vi "Test50.vi"(0 "L2T":T1 caption="Limites de test pris en compte", 2 "SN":string="0B5MEVA000CA1JC1M0000041", 3 "errin":errorcluster, 5 "Peak":T2=enum."PCAN_USBBUS1") -> (7 "RequetSQL":string, 8 "v1":string, 10 "errout":errorcluster)   [LabVIEW 2020]
uses:
  <userlib>/PCAN Basic/Controls/Channel.ctl
  Ctrl/L2T.ctl
  VarGLO/Global var.vi
  <vilib>/regexp/Match Regular Expression.xnode
  <userlib>/PCAN Basic/PCANBasic.lvlib
panel:
  out "cluster de sortie":T3
  # "Pre DCIR_____________________________________"
  # "intra DCIR_____________________________________"
  # "Post DCIR_____________________________________"
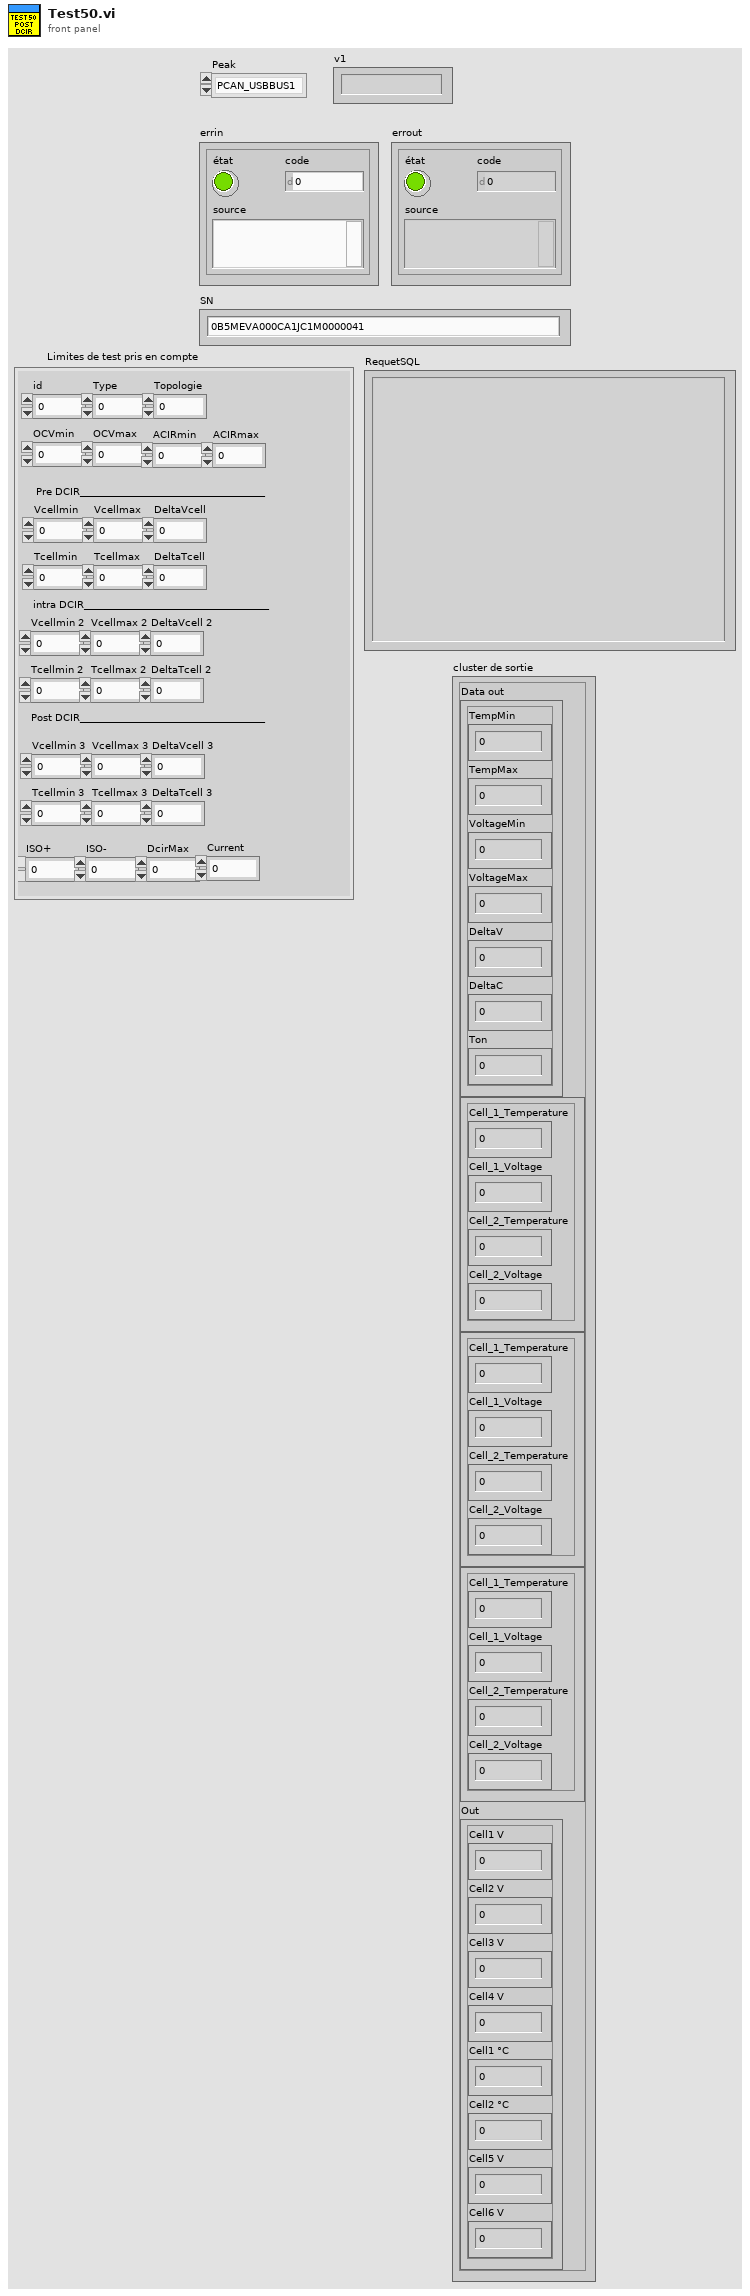
[diagram p1: front panel]
types:
  T1 = typedef "L2T.ctl" = cluster{"id":dbl, "Type":dbl, "OCVmin":dbl, "OCVmax":dbl, "ACIRmin":dbl, "ACIRmax":dbl, "Vcellmin":dbl, "Vcellmax":dbl, "DeltaVcell":dbl, "Tcellmin":dbl, "Tcellmax":dbl, "DeltaTcell":dbl, "ISO+":dbl, "ISO-":dbl, "DcirMax":dbl, "Current":dbl, "Topologie":dbl, "Vcellmin 2":dbl, "Vcellmax 2":dbl, "DeltaVcell 2":dbl, "Tcellmin 2":dbl, "Tcellmax 2":dbl, "DeltaTcell 2":dbl, "Vcellmin 3":dbl, "Vcellmax 3":dbl, "DeltaVcell 3":dbl, "Tcellmin 3":dbl, "Tcellmax 3":dbl, "DeltaTcell 3":dbl}
  T2 = typedef "PCANBasic.lvlib/Channel.ctl" = enum16{"PCAN_NONEBUS", "not used1", "not used2", "not used3", "not used4", "not used5", "not used6", "not used7", "not used8", "not used9", "not used10", "not used11", "not used12", "not used13", "not used14", "not used15", "not used16", "not used17", "not used18", "not used19", "not used20", "not used21", "not used22", "not used23", "not used24", "not used25", "not used26", "not used27", "not used28", "not used29", "not used30", "not used31", "not used32", "PCAN_ISABUS1", "PCAN_ISABUS2", "PCAN_ISABUS3", "PCAN_ISABUS4", "PCAN_ISABUS5", "PCAN_ISABUS6", "PCAN_ISABUS7", "PCAN_ISABUS8", "not used41", "not used42", "not used43", "not used44", "not used45", "not used46", "not used47", "not used48", "PCAN_DNGBUS1", "not used50", "not used51", "not used52", "not used53", "not used54", "not used55", "not used56", "not used57", "not used58", "not used59", "not used60", "not used61", "not used62", "not used63", "not used64", "PCAN_PCIBUS1", "PCAN_PCIBUS2", "PCAN_PCIBUS3", "PCAN_PCIBUS4", "PCAN_PCIBUS5", "PCAN_PCIBUS6", "PCAN_PCIBUS7", "PCAN_PCIBUS8", "not used73", "not used74", "not used75", "not used76", "not used77", "not used78", "not used79", "not used80", "PCAN_USBBUS1", "PCAN_USBBUS2", "PCAN_USBBUS3", "PCAN_USBBUS4", "PCAN_USBBUS5", "PCAN_USBBUS6", "PCAN_USBBUS7", "PCAN_USBBUS8", "Not used89", "Not used90", "Not used91", "Not used92", "Not used93", "Not used94", "Not used95", "Not used96", "PCAN_PCCBUS1", "PCAN_PCCBUS2"}
  T3 = cluster{"Data out":cluster{"TempMin":sgl, "TempMax":sgl, "VoltageMin":sgl, "VoltageMax":sgl, "DeltaV":sgl, "DeltaC":sgl, "Ton":sgl}, "Cluster":cluster{"Cell_1_Temperature":sgl, "Cell_1_Voltage":sgl, "Cell_2_Temperature":sgl, "Cell_2_Voltage":sgl}, "Cluster":cluster{"Cell_1_Temperature":sgl, "Cell_1_Voltage":sgl, "Cell_2_Temperature":sgl, "Cell_2_Voltage":sgl}, "Cluster":cluster{"Cell_1_Temperature":sgl, "Cell_1_Voltage":sgl, "Cell_2_Temperature":sgl, "Cell_2_Voltage":sgl}, "Out":cluster{"Cell1 V":sgl, "Cell2 V":sgl, "Cell3 V":sgl, "Cell4 V":sgl, "Cell1 °C":sgl, "Cell2 °C":sgl, "Cell5 V":sgl, "Cell6 V":sgl}}
  T4 = cluster{"Cell1 V":sgl, "Cell2 V":sgl, "Cell3 V":sgl, "Cell4 V":sgl, "Cell1 °C":sgl, "Cell2 °C":sgl, "Cell5 V":sgl, "Cell6 V":sgl}
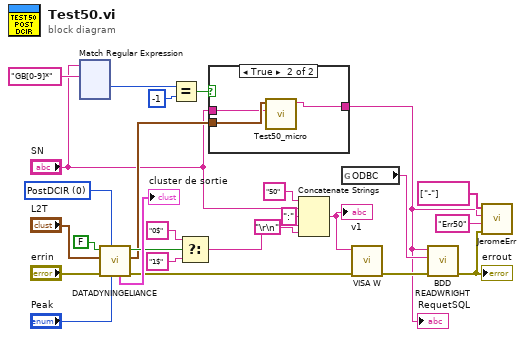
[diagram p0: block diagram]
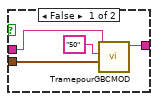
[diagram p2: hidden frame]
diagram:
  w1 = u16 0 items=["PostDCIR", "intraDCIR", "PreDCIR"] ("StepCMOD")
  n1 = xnode "Match Regular Expression"("input string"="SN", "regular expression"="GB[0-9]*") -> ("offset past match"=w9:i32)  [unwired: 4 in, 4 out]
  n2 = call "DATADYNINGELIANCE.vi"("Channel"="Peak", "StepCMOD"=w1, "errin"="errin", "L2T"="L2T", "3P4S"=FALSE) -> ("errout"=w13:errorcluster, "Out"=w6:T4, "test OK?"=w16:bool, "cluster de sortie"=→"cluster de sortie":T3)  [unwired: 2 in, 1 out]
  n3 = Equal?(x=w9, y=-1) -> (x = y?=w3:bool)
  n4 = Select(t="0$" ("chaîne"), s=w16, f="1$" ("chaîne")) -> (s? t:f=w22:string)
  n5 = case shown="True" w3 {
    tunnel: w6 -> [w30 w34]
    tunnel: "SN" -> [w28 w33]
    tunnel: [w29 w32] -> w4
    frame False {
      n6 = call "TramepourGBCMOD.vi"("Out"=w30, "TestNum"="50", "SN"=w28) -> ("String"=w29:string)  [unwired: 8 in]
    }
    frame True {
      n7 = call "Test50_micro.vi"("SN"=w33, "Out"=w34) -> ("String"=w32:string)  [unwired: 8 in]
    }
  }
  "RequetSQL" <- w4
  n8 = Concatenate Strings("50" ("chaîne"), "SN", ":" ("string"), w22, "\r\n") -> (w11:string)
  "v1" <- w11
  n9 = global read "Global var.vi" "ODBC"() -> (w7:string)
  n10 = call "VISA W.vi"("errin"=w13, "Chaîne"=w11) -> ("errout"=w12:errorcluster)  [unwired: 9 in]
  n11 = call <userlib>:"BDD READWRIGHT.vi"("errin"=w12, "DSN name"=w7, "Instruction"=w4) -> ("error out"=w14:errorcluster)  [unwired: 7 in, 1 out]
  "errout" <- w14
  n12 = call "JeromeErr.vi"("Errin"=w14, "CodeERR"="Err50", "RequetteSQL"=w4, "RetourSQL"=string[] ["-"]) -> ()  [unwired: 8 in]
